vi "STFT vs RPM (analog).vi"(0 "scaled signal [EU]":dbl[](array[numeric]) format="%.2f", 1 "tacho signal [V]":dbl[](array[numeric]) format="%.2f", 2 "sampling frequency [Hz]":dbl=10000.0 format="%.2f", 3 "rpm segment":T1={"from [rpm]"=2000.0, "to [rpm]"=4000.0, "rpm increment [rpm]"=100.0} {"rpm increment [rpm]" min=1.0 format="%.2f"; "to [rpm]" format="%.2f"; "from [rpm]" format="%.2f"}, 4 "tacho info":T2={"threshold [V]"=1.0, "pulse width (2)"=2, "avg on n pulses (2)"=2, "pulse/revolution (1)"=1} {"pulse/revolution (1)" min=1 step=1; "avg on n pulses (2)" min=2 step=1; "pulse width (2)" min=1; "threshold [V]" format="%.2f"}, 5 "channel info":T3={"sensor sensitivity [mV/EU]"=1000.0, "engineering units"=enum."V", "dB reference [EU]"=1.0, "custom label"="EU", "weighting filter"=enum."Linear", "pregain [dB]"=0.0} {"dB reference [EU]" format="%.1e"; "pregain [dB]" format="%.2f"; "sensor sensitivity [mV/EU]" format="%.2f"}, 6 "window":T4 items=["Rectangle"=0, "Hanning"=1, "Hamming"=2, "Blackman-Harris"=3, "Exact Blackman"=4, "Blackman"=5, "Flat Top"=6, "4 Term B-Harris "=7, "7 Term B-Harris"=8, "Low Sidelobe"=9, "Blackman Nuttall"=11, "Triangle"=30, "Bartlett-Hanning"=31, "Bohman"=32, "Parzen"=33, "Welch"=34, "Kaiser"=60, "Dolph-Chebyshev"=61, "Gaussian"=62], 7 "FFT block size":i32=1024 min=1, 8 "frequency weighting":T5(ring), 9 "dB On (T)":bool=TRUE) -> (14 "power spectrum [EU^2 rms]":dbl[][](array[numeric]) format="%.2f", 15 "unit label":string, 16 "rpm0 and delta rpm [rpm]":cluster{"rpm0":dbl, "delta rpm":dbl} {"delta rpm" format="%.2f"; "rpm0" format="%.2f"}, 17 "f0 and delta f [Hz]":cluster{"f0":dbl, "delta f":dbl} {"delta f" format="%.2f"; "f0" format="%.2f"}, 18 "rpm vs. time":cluster{"time [s]":dbl[], "speed [rpm]":dbl[]} {"speed [rpm]" format="%.2f"; "time [s]" format="%.2f"}, 19 "weighting conflict":bool)   [LabVIEW 2017]
doc: "Performs an STFT (Short-Time Fourier Transform) on the input signal as a function of the rotational speed recorded by tacho signal.\nThe rpm segment cluster specifies the revolutions per minute range to analyze (low and high revolutions per minute) and the revolutions per minute increment.\nThe tacho info cluster specifies the characteristics of the pulses generated by the tachometer (threshold and pulse width), the number of pulses per revolution, and the number of pulses used to compute the rotational speed.\nThis VI returns a 2D array that contains the power spectrum at the various selected rotational speeds. The VI returns evolution of the rotational speed (revolutions per minute) as a function of time and the information (rpm0 and delta rpm, f0 and delta f) needed to display the results on a colormap or a waterfall display."
uses:
  <vilib>/Analysis/4window.llb/windowTd.ctl
  <vilib>/Analysis/NI_AALPro.lvlib
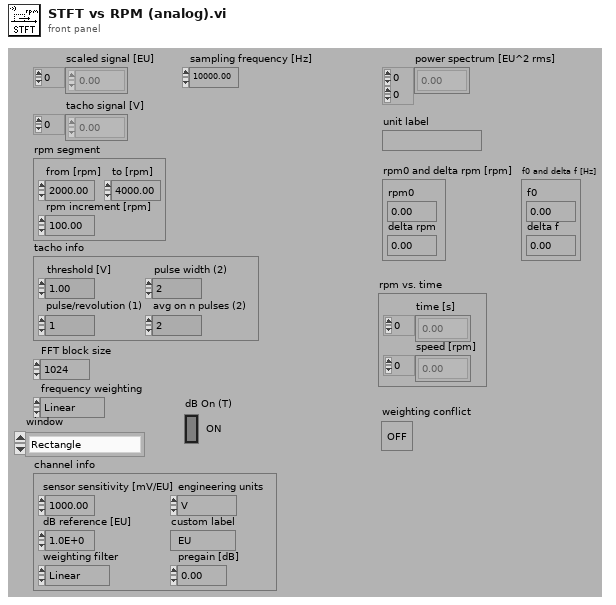
[diagram p1: front panel]
types:
  T1 = cluster{"from [rpm]":dbl, "to [rpm]":dbl, "rpm increment [rpm]":dbl}
  T2 = cluster{"threshold [V]":dbl, "pulse width (2)":i32, "avg on n pulses (2)":i32, "pulse/revolution (1)":i32}
  T3 = cluster{"sensor sensitivity [mV/EU]":dbl, "engineering units":enum16{"custom...", "V", "Pa", "g", "m/s^2", "m/s", "m", "in/s^2", "in/s", "in"}, "dB reference [EU]":dbl, "custom label":string, "weighting filter":enum16{"Linear", "A-weighting", "B-weighting", "C-weighting"}, "pregain [dB]":dbl}
  T4 = typedef "NI_AALPro.lvlib/windowTd.ctl" = u32
  T5 = enum16{"Linear", "A-weighting", "B-weighting", "C-weighting"}
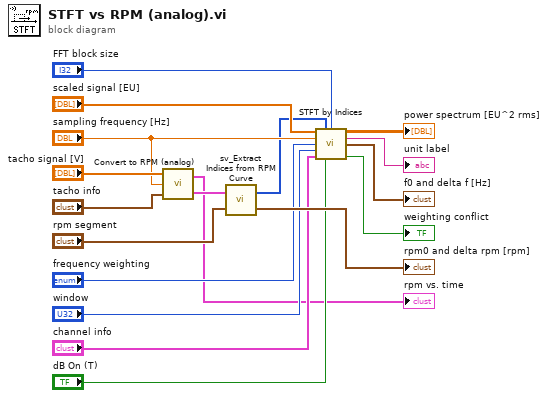
[diagram p0: block diagram]
diagram:
  n1 = call <vilib>:"Convert to RPM (analog).vi"("tacho info"="tacho info", "sampling frequency [Hz]"="sampling frequency [Hz]", "tacho signal [V]"="tacho signal [V]") -> ("rpm vs. indices"=w17:cluster{"indices":dbl[], "speed [rpm]":dbl[]}, "rpm vs. time"=→"rpm vs. time":cluster{"time [s]":dbl[], "speed [rpm]":dbl[]})
  n2 = call <vilib>:"sv_Extract Indices from RPM Curve.vi"("rpm segment"="rpm segment", "rpm vs. indices"=w17) -> ("rpm0 and delta rpm [rpm]"=→"rpm0 and delta rpm [rpm]":cluster{"rpm0":dbl, "delta rpm":dbl}, "indices"=w12:i32[])
  n3 = call <vilib>:"STFT by Indices.vi"("scaled signal [EU]"="scaled signal [EU]", "indices"=w12, "FFT block size"="FFT block size", "sampling frequency [Hz]"="sampling frequency [Hz]", "frequency weighting"="frequency weighting", "window"="window", "channel info"="channel info", "dB On (T)"="dB On (T)") -> ("power spectrum [EU^2 rms]"=→"power spectrum [EU^2 rms]":dbl[][], "unit label"=→"unit label":string, "f0 and delta f [Hz]"=→"f0 and delta f [Hz]":cluster{"f0":dbl, "delta f":dbl}, "weighting conflict"=→"weighting conflict":bool)  [unwired: 4 in]
